vi "Available I2C.vi"(8 "error in (no error)":errorcluster, 11 "DeviceComms in":refnum<class "DeviceComms.lvclass">) -> (0 "error out":errorcluster, 2 "Available I2C":T1[](array[typedef]), 3 "DeviceComms out":refnum<class "DeviceComms.lvclass">)   [LabVIEW 2020, in "CTI.lvlib" / "DeviceComms.lvclass"]
uses:
  DeviceComms.lvclass
  GPIO Number.ctl
  CTI.lvlib
  I2C Number.ctl
  Available I2C.ctl
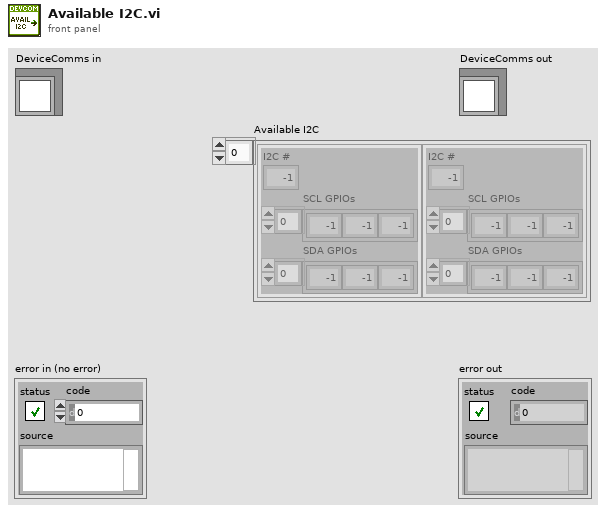
[diagram p1: front panel]
types:
  T1 = typedef "CTI.lvlib/Available I2C.ctl" = cluster{"I2C #":T2, "SCL GPIOs":T3[], "SDA GPIOs":T3[]}
  T2 = typedef "CTI.lvlib/I2C Number.ctl" = i8
  T3 = typedef "CTI.lvlib/GPIO Number.ctl" = i8
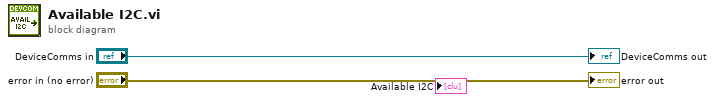
[diagram p0: block diagram]
diagram:
  "error out" <- "error in (no error)"
  "DeviceComms out" <- "DeviceComms in"
